vi "ListenerForMotion.vi"(10 "UIMsg":T1, 11 "UI Messages":string) -> (3 "String":string)   [LabVIEW 2017]
uses:
  Support/MessageAPI/UIMessage.ctl
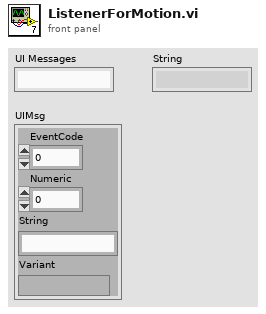
[diagram p1: front panel]
types:
  T1 = typedef "UIMessage.ctl" = cluster{"EventCode":i32, "Numeric":dbl, "String":string, "Variant":variant}
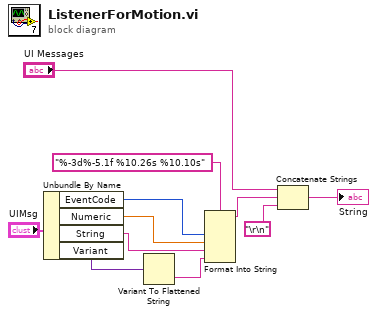
[diagram p0: block diagram]
diagram:
  n1 = Unbundle By Name("UIMsg") -> ("EventCode"=w3:i32, "Numeric"=w8:dbl, "String"=w7:string, "Variant"=w5:variant)
  n2 = Variant To Flattened String(Variant=w5) -> (data string=w6:string)  [unwired: 1 out]
  n3 = Format Into String(format string="%-3d%-5.1f %10.26s %10.10s", w3, w8, w7, w6) -> (resulting string=w9:string)  [unwired: 2 in, 1 out]
  n4 = Concatenate Strings("UI Messages", w9, "\r\n") -> (→"String":string)
